vi "__ABB start.vi"() -> ()   [LabVIEW 2017]
uses:
  ABB global.vi
panel:
  in  "stop":bool
  in  "Continue Test":bool
  in  "View Test":bool
  in  "Enter":bool
  in  "Password":string caption="Type in Password, \nthen press 'Enter'"
  in  "New Test":bool
  in  "Configure":bool
  in  "Quit":bool
  # "MOTOR TEST"
  # "Version 3.92"
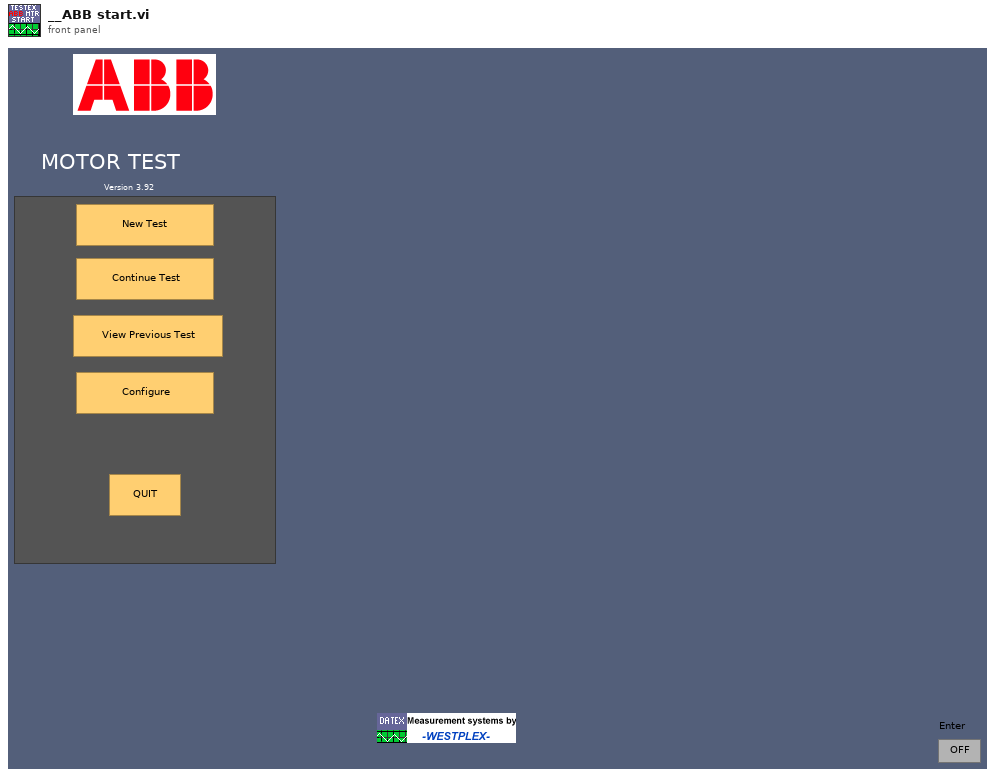
[diagram p1: front panel]
types:
  T1 = enum32{"existing file", "new file", "new or existing file", "existing dir", "new dir", "new or existing dir", "existing file (use LLBs)", "new file (use LLBs)", "new or existing file (use LLBs)", "new or existing file or directory (use LLBs)"}
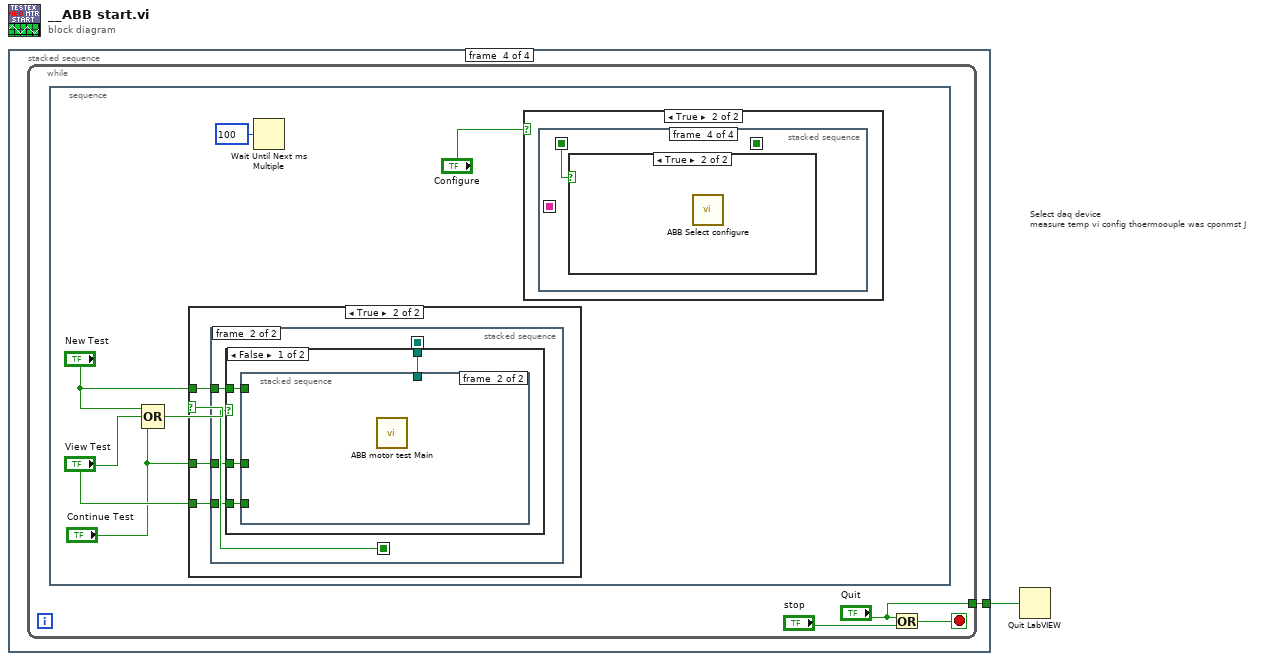
[diagram p0: block diagram]
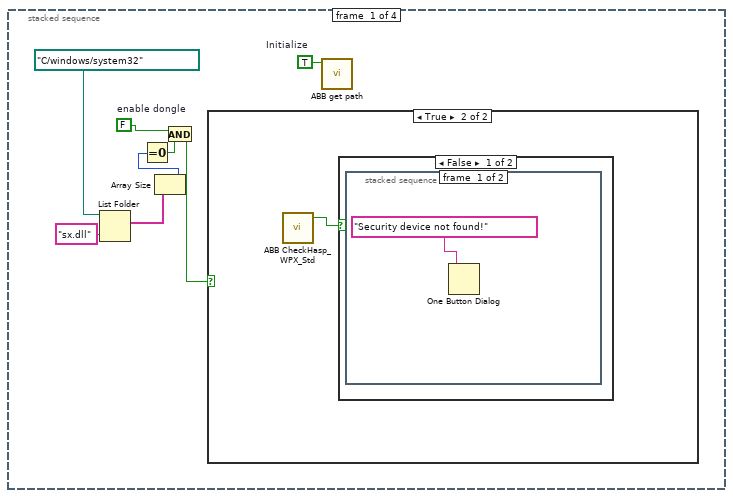
[diagram p2: hidden frame]
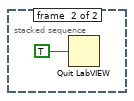
[diagram p4: hidden frame]
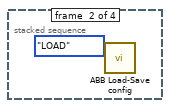
[diagram p6: hidden frame]
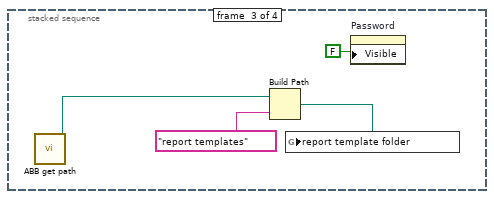
[diagram p7: hidden frame]
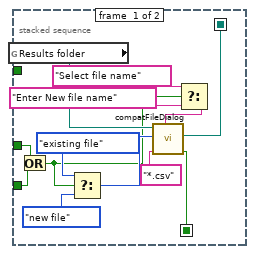
[diagram p9: hidden frame]
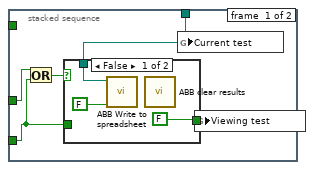
[diagram p10: hidden frame]
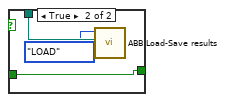
[diagram p11: hidden frame]
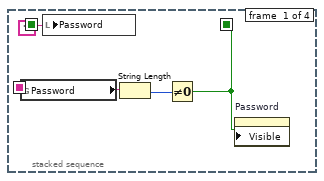
[diagram p14: hidden frame]
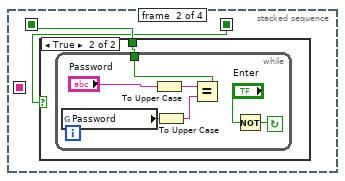
[diagram p15: hidden frame]
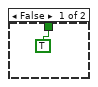
[diagram p16: hidden frame]
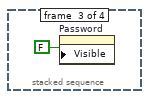
[diagram p17: hidden frame]
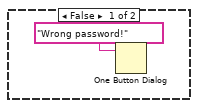
[diagram p18: hidden frame]
diagram:
  # "Select daq device\nmeasure temp vi config thoermoouple was cponmst J"
  n1 = stacked-sequence {
    tunnel: [_ _ _ w18] -> w1
    frame #0 {
      w2 = TRUE  # Initialize
      w5 = FALSE  # enable dongle
      n2 = List Folder(path=path "C:/windows/system32", pattern="sx.dll") -> (filenames=w8:string[])  [unwired: 2 in, 3 out]
      n3 = Array Size(array=w8) -> (size(s)=w7:i32)
      n4 = Equal To 0?(x=w7) -> (x = 0?=w6:bool)
      n5 = And(x=w5, y=w6) -> (x .and. y?=w3:bool)
      n6 = case shown="True" w3 {
        frame False {
        }
        frame True {
          n7 = call "ABB CheckHasp_WPX_Std.vi"() -> ("Verified"=w10:bool)  [unwired: 11 in]
          n8 = case shown="False" w10 {
            frame False {
              n9 = stacked-sequence {
                frame #0 {
                  n10 = One Button Dialog(message="Security device not found!") -> ()  [unwired: 1 in, 1 out]
                }
                frame #1 {
                  n11 = Quit LabVIEW(quit? (T)=TRUE) -> ()
                }
              }
            }
            frame True {
            }
          }
        }
      }
      n12 = call "ABB get path.vi"("Initialize"=w2) -> ()  [unwired: 10 in, 1 out]
    }
    frame #1 {
      n13 = call "ABB Load-Save config.vi"("Mode"=enum16{"LOAD", "SAVE"}."LOAD") -> ()  [unwired: 11 in]
    }
    frame #2 {
      n14 = call "ABB get path.vi"() -> ("Path"=w14:path)  [unwired: 11 in]
      n15 = Build Path(base path=w14, name or relative path="report templates") -> (appended path=w16:path)
      n16 = global write "ABB global.vi" "report template folder"(w16) -> ()
      n17 = property on="Password" class="Str"("Visible"=FALSE) -> ()  [unwired: 2 in, 2 out]
    }
    frame #3 {
      n18 = while {
        tunnel: ["Quit"] -> w18
        stop <- w21 stop-if-true
        n19 = stacked-sequence {
          frame #0 {
            n20 = Compound Arithmetic op=OR("New Test", "View Test", "Continue Test") -> (w25:bool)
            n21 = case shown="True" w25 {
              tunnel: "View Test" -> [_ w30]
              tunnel: "Continue Test" -> [_ w29]
              tunnel: "New Test" -> [_ w28]
              frame False {
              }
              frame True {
                n22 = stacked-sequence {
                  seq-local: [w41 _] -> [_ w47]
                  seq-local: [w40 _] -> [_ w48]
                  tunnel: w30 -> [w34 w46]
                  tunnel: w29 -> [w32 w45]
                  tunnel: w28 -> [_ w44]
                  frame #0 {
                    n23 = global read "ABB global.vi" "Results folder"() -> (w42:path)
                    n24 = Or(x=w32, y=w34) -> (x .or. y?=w31:bool)
                    n25 = Select(t=T1."existing file", s=w31, f=T1."new file" ("select mode (2)")) -> (s? t:f=w38:T1)
                    n26 = Select(t="Select file name", s=w31, f="Enter New file name" ("prompt")) -> (s? t:f=w35:string)
                    n27 = call <vilib>:"compatFileDialog.vi"("prompt"=w35, "pattern"="*.csv", "select mode (2)"=w38, "start path"=w42) -> ("cancelled"=w40:bool, "path"=w41:path)  [unwired: 5 in, 1 out]
                  }
                  frame #1 {
                    n28 = case shown="False" w48 {
                      tunnel: w47 -> [w52 _]
                      tunnel: w46 -> [w51 _]
                      tunnel: w45 -> [w50 _]
                      tunnel: w44 -> [w49 _]
                      frame False {
                        n29 = stacked-sequence {
                          tunnel: w52 -> [w57 _]
                          tunnel: w51 -> [w53 _]
                          tunnel: w50 -> [w54 _]
                          tunnel: w49 -> [_ _]
                          frame #0 {
                            n30 = Or(x=w54, y=w53) -> (x .or. y?=w55:bool)
                            n31 = case shown="False" w55 {
                              tunnel: w57 -> [w60 w63]
                              tunnel: [FALSE w61] -> w56
                              tunnel: w53 -> [_ w61]
                              frame False {
                                n32 = call "ABB Write to spreadsheet.vi"("append to file? (new file:F)"=FALSE, "file path (dialog if empty)"=w60) -> ()  [unwired: 6 in, 1 out]
                                n33 = call "ABB clear results.vi"() -> ()  [unwired: 1 in]
                              }
                              frame True {
                                n34 = call "ABB Load-Save results.vi"("Path"=w63, "Mode"=enum16{"LOAD", "Save"}."LOAD") -> ()  [unwired: 10 in]
                              }
                            }
                            n35 = global write "ABB global.vi" "Current test"(w57) -> ()
                            n36 = global write "ABB global.vi" "Viewing test"(w56) -> ()
                          }
                          frame #1 {
                            n37 = call "ABB motor test Main.vi"() -> ()  [unwired: 1 in]
                          }
                        }
                      }
                      frame True {
                      }
                    }
                  }
                }
              }
            }
            n38 = Wait Until Next ms Multiple(millisecond multiple=u32 100) -> ()  [unwired: 1 out]
            n39 = case shown="True" "Configure" {
              frame False {
              }
              frame True {
                n40 = stacked-sequence {
                  seq-local: [_ w69 _ _] -> [_ _ _ w80]
                  seq-local: [w66 _ _ _] -> [_ _ _ _]
                  seq-local: [w64 _ _ _] -> [_ w68 _ _]
                  frame #0 {
                    n41 = global read "ABB global.vi" "Password"() -> (w66:string)
                    n42 = local write "Password"("") -> ()
                    n43 = String Length(string=w66) -> (length=w65:i32)
                    n44 = Not Equal To 0?(x=w65) -> (x != 0?=w64:bool)
                    n45 = property on="Password" class="Str"("Visible"=w64) -> ()  [unwired: 2 in, 2 out]
                  }
                  frame #1 {
                    n46 = case shown="True" w68 {
                      tunnel: [TRUE w71] -> w69
                      frame False {
                      }
                      frame True {
                        n47 = while {
                          tunnel: [w76] -> w71
                          stop <- w77 continue-if-true
                          n48 = global read "ABB global.vi" "Password"() -> (w78:string)
                          n49 = To Upper Case(1:"Password") -> (0:w74:string)
                          n50 = To Upper Case(1:w78) -> (0:w73:string)
                          n51 = Equal?(x=w74, y=w73) -> (x = y?=w76:bool)
                          n52 = Not(x="Enter") -> (.not. x?=w77:bool)
                        }
                      }
                    }
                  }
                  frame #2 {
                    n53 = property on="Password" class="Str"("Visible"=FALSE ("Write Attribute")) -> ()  [unwired: 2 in, 2 out]
                  }
                  frame #3 {
                    n54 = case shown="True" w80 {
                      frame False {
                        n55 = One Button Dialog(message="Wrong password!") -> ()  [unwired: 1 in, 1 out]
                      }
                      frame True {
                        n56 = call "ABB Select configure.vi"() -> ()  [unwired: 12 in]
                      }
                    }
                  }
                }
              }
            }
          }
        }
        n57 = Or(x="Quit", y="stop") -> (x .or. y?=w21:bool)
      }
    }
  }
  n58 = Quit LabVIEW(quit? (T)=w1) -> ()
